vi "to-string.vi"(8 "error in (no error)":errorcluster, 11 "G.lvlib:ID.lvclass":refnum<class "ID.lvclass">) -> (0 "error out":errorcluster, 2 "string":string, 3 "G.lvlib:ID.lvclass":refnum<class "ID.lvclass">)   [LabVIEW 2020, in "graph.lvlib" / "ID.lvclass"]
uses:
  ID.lvclass
  ID.lvclass/ID.ctl
  support/UUID/UUID.lvclass
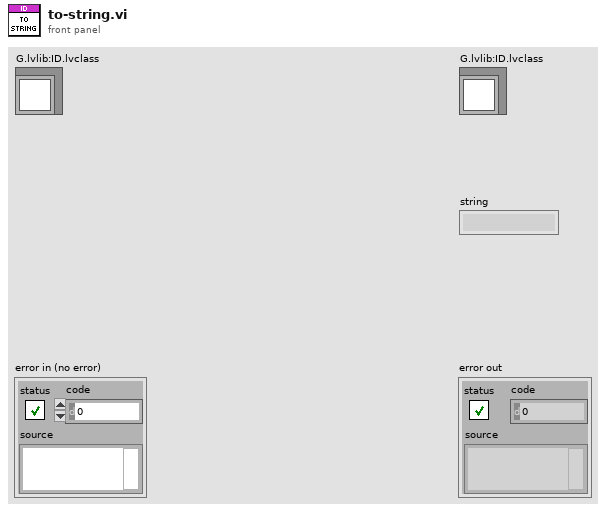
[diagram p1: front panel]
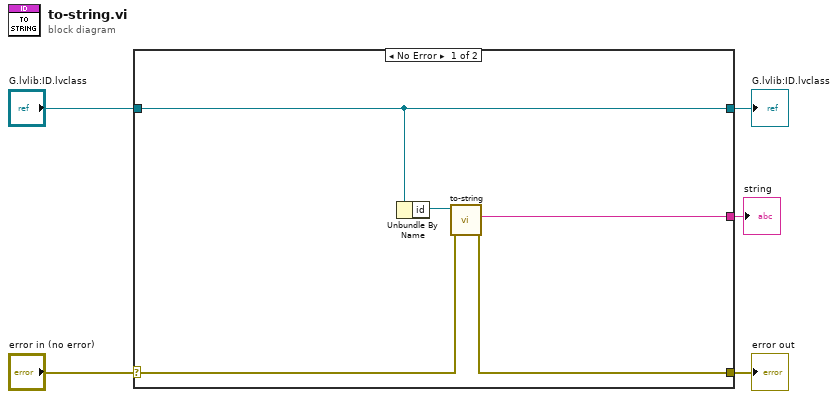
[diagram p0: block diagram]
diagram:
  n1 = case shown="No Error" "error in (no error)" {
    selector: "error in (no error)" -> [w7 w12]
    tunnel: [w6 w12] -> w4
    tunnel: [w10 w11] -> w2
    tunnel: "G.lvlib:ID.lvclass" -> [w10 w11]
    tunnel: [w8 _] -> w1
    frame No Error {
      n2 = Unbundle By Name(w10) -> ("id"=w9:refnum<class "UUID.lvclass">)
      n3 = call "to-string.vi"("error in (no error)"=w7, "UUID in"=w9) -> ("error out"=w6:errorcluster, "uuid-string"=w8:string)  [unwired: 8 in]
    }
    frame Error {
    }
  }
  "error out" <- w4
  "G.lvlib:ID.lvclass" <- w2
  "string" <- w1
